vi "Insert Nested Sequences Recursivly.vi"(6 "Inserted Sequence Name Array":string[](array[string]), 7 "Message List Elements":T4[](array[typedef]), 8 "error in (no error)":errorcluster, 9 "Sequence folder path":path, 10 "Override Look up table in":variant, 11 "Uncompiled sequence in":T1[](array[typedef])) -> (0 "error out":errorcluster, 2 "Override Look up table out":variant, 3 "Uncompiled Sequence out":T1[](array[typedef]))   [LabVIEW 2020, in "Sequencer.lvlib"]
doc: "Recursivly load and insert Uncompiled Sequences replacing all Nested Sequence Msgs."
uses:
  Sequencer.lvlib
  Controls/Ctl_MessageListElement.ctl
  Controls/Ctl_SequenceElement.ctl
  Controls/Ctl_SequenceControlElement.ctl
  PPL/HDH.Actor Framework.Core.Msg.lvlibp/Flex Msg/Controls/Ctl_Control Element.ctl
  Sequencer Messages/Nested Sequence Msg/Nested Sequence Msg.lvclass
  Sequencer Messages/Nested Sequence Msg/Controls/Ctl_SequenceNameArrayCluster.ctl
  PPL/HDH.Data.Generic.lvlibp
  PPL/HDH.Actor Framework.Core.Msg.lvlibp
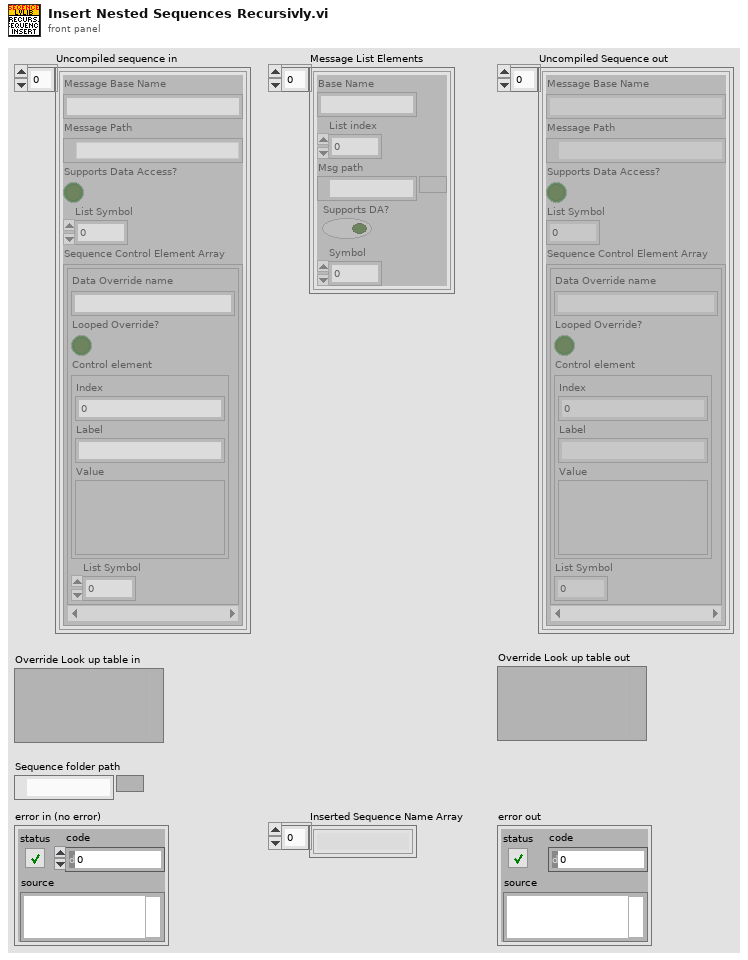
[diagram p1: front panel]
types:
  T1 = typedef "Sequencer.lvlib/Ctl_SequenceElement.ctl" = cluster{"Message Base Name":string, "Message Path":path, "Supports Data Access?":bool, "List Symbol":i32, "Sequence Control Element Array":T2[]}
  T2 = typedef "Sequencer.lvlib/Ctl_SequenceControlElement.ctl" = cluster{"Data Override name":string, "Looped Override?":bool, "Control element":T3, "List Symbol":i32}
  T3 = typedef "HDH.Actor Framework.Core.Msg.lvlibp/Ctl_Control Element.ctl" = cluster{"Index":i32, "Label":string, "Value":variant}
  T4 = typedef "Sequencer.lvlib/Ctl_MessageListElement.ctl" = cluster{"Base Name":string, "List index":i32, "Msg path":path, "Supports DA?":bool, "Symbol":i32}
  T5 = typedef "Sequencer.lvlib/Nested Sequence Msg.lvclass/Ctl_SequenceNameArrayCluster.ctl" = cluster{"Sequence Name Array":string[]}
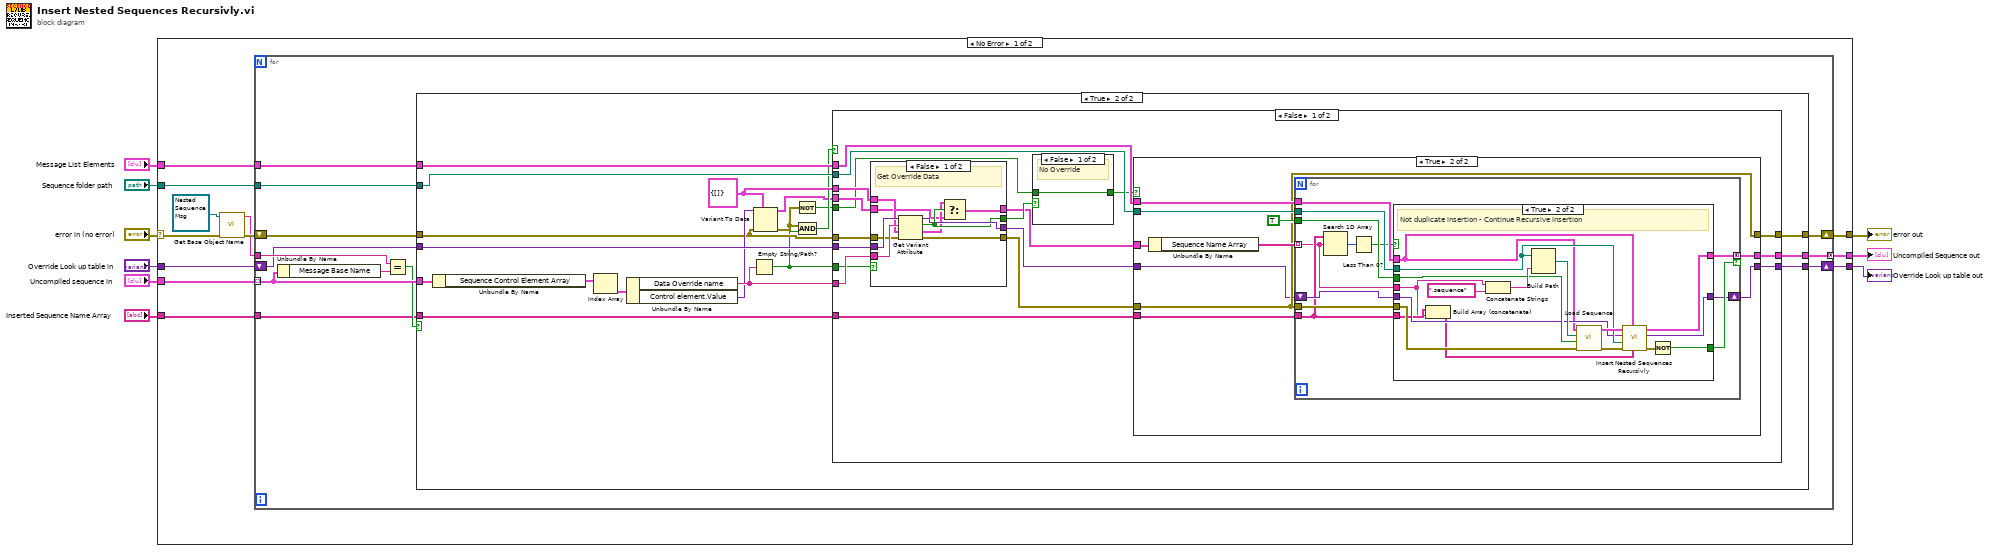
[diagram p0: block diagram]
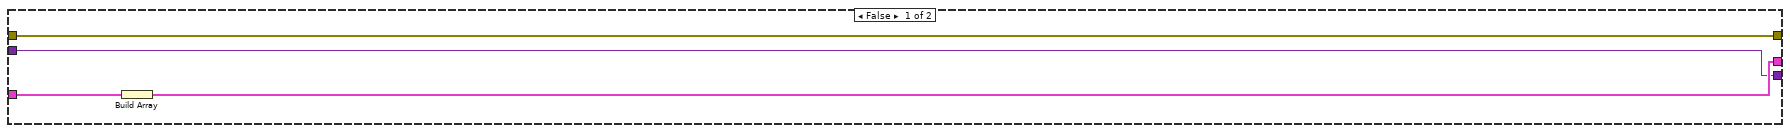
[diagram p2: hidden frame]
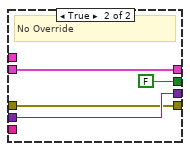
[diagram p4: hidden frame]
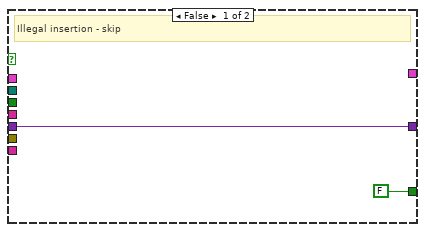
[diagram p6: hidden frame]
diagram:
  n1 = case shown="No Error" "error in (no error)" {
    selector: "error in (no error)" -> [w18 w137]
    tunnel: "Message List Elements" -> [w17 _]
    tunnel: "Sequence folder path" -> [w16 _]
    tunnel: "Override Look up table in" -> [w15 w136]
    tunnel: [w14 w136] -> w5
    tunnel: [w13 w137] -> w4
    tunnel: [w12 _] -> w3
    tunnel: "Uncompiled sequence in" -> [w11 _]
    tunnel: "Inserted Sequence Name Array" -> [w10 _]
    frame No Error {
      n2 = call "Get Base Object Name.vi"("error in (no error)"=w18, "Object in"=refnum<class "Nested Sequence Msg.lvclass"> refnum ("Sequencer.lvlib:Nested Sequence Msg.lvclass")) -> ("error out"=w21:errorcluster, "Base class name"=w20:string)  [unwired: 8 in]
      n3 = for {
        tunnel: w11 -> [w32] mode=indexing
        tunnel: [w33] -> w12 mode=concatenating
        tunnel: w20 -> [w30]
        shift-right: [w29] -> w13
        shift-left: w21 -> [w28]
        shift-right: [w27] -> w14
        shift-left: w15 -> [w26]
        tunnel: w16 -> [w25]
        tunnel: w17 -> [w24]
        tunnel: w10 -> [w22]
        n4 = Unbundle By Name(w32) -> ("Message Base Name"=w31:string)
        n5 = Equal?(x=w30, y=w31) -> (x = y?=w23:bool)
        n6 = case shown="True" w23 {
          tunnel: [w37 w47] -> w33
          tunnel: w32 -> [w36 w56]
          tunnel: [w35 w50] -> w29
          tunnel: w28 -> [w35 w42]
          tunnel: [w34 w52] -> w27
          tunnel: w26 -> [w34 w53]
          tunnel: w25 -> [_ w49]
          tunnel: w24 -> [_ w48]
          tunnel: w22 -> [_ w46]
          frame False {
            n7 = Build Array(w36) -> (w37:T1[])
          }
          frame True {
            w45 = T5 {"Sequence Name Array"=[]} ("Sequence Name Array Cluster")
            n8 = Unbundle By Name(w56) -> ("Sequence Control Element Array"=w55:T2[])
            n9 = Index Array(array=w55) -> (element=w54:T2)  [unwired: 1 in]
            n10 = Unbundle By Name(w54) -> ("Data Override name"=w51:string, "Control element.Value"=w44:variant)
            n11 = Empty String/Path?(string/path=w51) -> (empty?=w41:bool)
            n12 = Variant To Data(error in=w42, type=w45, Variant=w44) -> (data=w40:T5, error out=w39:errorcluster)
            n13 = Not(x=w39) -> (.not. x?=w38:bool)
            n14 = And(x=w39, y=w41) -> (x .and. y?=w43:bool)
            n15 = case shown="False" w43 {
              tunnel: w53 -> [w74 w135]
              tunnel: [w65 w135] -> w52
              tunnel: w51 -> [w73 _]
              tunnel: [w67 w134] -> w50
              tunnel: w42 -> [w72 w134]
              tunnel: w49 -> [w71 _]
              tunnel: w48 -> [w70 _]
              tunnel: [w69 _] -> w47
              tunnel: w46 -> [w64 _]
              tunnel: w45 -> [w63 _]
              tunnel: w41 -> [w62 _]
              tunnel: w40 -> [w61 _]
              tunnel: w38 -> [w59 _]
              frame False {
                n16 = case shown="False" w62 {
                  tunnel: w74 -> [w86 w90]
                  tunnel: w73 -> [w85 _]
                  tunnel: [w80 FALSE] -> w60
                  tunnel: w72 -> [w84 w87]
                  tunnel: [w78 w88] -> w57
                  tunnel: [w83 w87] -> w68
                  tunnel: [w82 w90] -> w66
                  tunnel: w63 -> [w81 _]
                  tunnel: w61 -> [w77 w88]
                  frame False {
                    # "Get Override Data"
                    n17 = Get Variant Attribute(Variant=w86, name=w85, default value (empty Variant)=w81, error in=w84) -> (duplicate Variant=w82:variant, found=w80:bool, value=w79:T5, error out=w83:errorcluster)
                    n18 = Select(t=w79, s=w80, f=w77) -> (s? t:f=w78:T5)
                  }
                  frame True {
                    # "No Override"
                  }
                }
                n19 = case shown="False" w60 {
                  selector: w60 -> [_ w76]
                  tunnel: w59 -> [w75 _]
                  tunnel: [w75 w76] -> w58
                  frame False {
                    # "No Override"
                  }
                  frame True {
                    # "Override Success"
                  }
                }
                n20 = case shown="True" w58 {
                  tunnel: w57 -> [_ w102]
                  tunnel: w71 -> [_ w100]
                  tunnel: w70 -> [_ w98]
                  tunnel: [_ w97] -> w69
                  tunnel: w68 -> [w92 w96]
                  tunnel: [w92 w96] -> w67
                  tunnel: [w91 w94] -> w65
                  tunnel: w66 -> [w91 w95]
                  tunnel: w64 -> [_ w93]
                  frame False {
                  }
                  frame True {
                    n21 = Unbundle By Name(w102) -> ("Sequence Name Array"=w101:string[])
                    n22 = for {
                      tunnel: w101 -> [w105] mode=indexing
                      tunnel: w100 -> [w110]
                      tunnel: TRUE ("Skip File Dialog?(F)") -> [w114]
                      tunnel: w98 -> [w107]
                      tunnel: [w111] -> w97 mode=concatenating if=w113
                      tunnel: w96 -> [w112]
                      shift-right: [w108] -> w94
                      shift-left: w95 -> [w109]
                      tunnel: w93 -> [w106]
                      n23 = Search 1D Array(1D array=w106, element=w105) -> (index of element=w104:i32)  [unwired: 1 in]
                      n24 = Less Than 0?(x=w104) -> (x < 0?=w103:bool)
                      n25 = case shown="True" w103 {
                        tunnel: w114 -> [_ w131]
                        tunnel: [FALSE w129] -> w113
                        tunnel: w112 -> [_ w128]
                        tunnel: [_ w126] -> w111
                        tunnel: w110 -> [_ w123]
                        tunnel: w109 -> [w116 w122]
                        tunnel: [w116 w121] -> w108
                        tunnel: w107 -> [_ w120]
                        tunnel: w106 -> [_ w118]
                        tunnel: w105 -> [_ w117]
                        frame False {
                          # "Illegal insertion - skip"
                        }
                        frame True {
                          # "Not duplicate insertion - Continue Recursive Insertion"
                          n26 = Build Array (concatenate)(w118, w117) -> (w119:string[])
                          n27 = Concatenate Strings(w117, ".sequence" ("string")) -> (w132:string)
                          n28 = Build Path(base path=w123, name or relative path=w132) -> (appended path=w130:path)
                          n29 = call "Load Sequence.vi"("error in (no error)"=w128, "Skip File Dialog?(F)"=w131, "Browse path"=w130, "Message List Elements"=w120) -> ("error out"=w125:errorcluster, "Uncompiled Sequence out"=w127:T1[])  [unwired: 6 in]
                          n30 = call "Insert Nested Sequences Recursivly.vi"("Inserted Sequence Name Array"=w119, "Message List Elements"=w120, "error in (no error)"=w125, "Sequence folder path"=w123, "Override Look up table in"=w122, "Uncompiled sequence in"=w127) -> ("error out"=w124:errorcluster, "Override Look up table out"=w121:variant, "Uncompiled Sequence out"=w126:T1[])  [unwired: 3 in]
                          n31 = Not(x=w124) -> (.not. x?=w129:bool)
                        }
                      }
                    }
                  }
                }
              }
              frame True {
                # "Neither Override nor regular data"
              }
            }
          }
        }
      }
    }
    frame Error {
    }
  }
  "Override Look up table out" <- w5
  "error out" <- w4
  "Uncompiled Sequence out" <- w3
